vi "Status Monitor (Single Unit).vi"(9 "Update Status Event":refnum<user-event>, 10 "Device Index":i32, 11 "configuration file path":path) -> ()   [LabVIEW 2017, in "Status Monitor Library.lvlib"]
doc: "Connects to the status port and frequently reads the buffer. \n\nAttempts to decode that data in a status message. If the decoding is sucessful, a user event is triggered and that status message is made available through the event."
uses:
  Status Monitor Library.lvlib
  Combined Status and Transient/SubVIs/Device Status and Index--Cluster.ctl
  Communications/Typedefs/DTACQ Module Carrier Status.ctl
  Communications/Typedefs/DTACQ Status--Enum.ctl
  Communications/Communications Library.lvlib
panel:
  in  "Stop":bool
  out "Demuxing":bool
  out "Total Samples":i32
  out "Post-Buffered Samples":i32
  out "Pre-Buffered Samples":i32
  out "Device State":T1(ring)
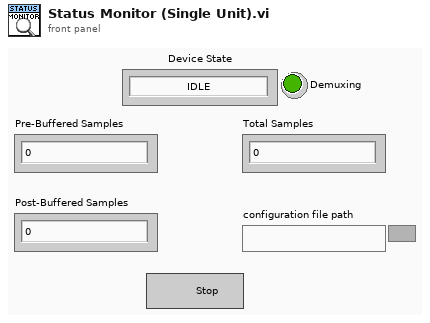
[diagram p1: front panel]
types:
  T1 = enum16{"IDLE", "ARM", "RUN_PRE-TRIGGER", "RUN_POST-TRIGGER", "POST_PROCESS", "CLEANUP"}
  T2 = typedef "Communications Library.lvlib/DTACQ Module Carrier Configuration--Cluster.ctl" = cluster{"Name":string, "IP":string, "Control Port":i32, "Timeout (ms)":i32, "Continuous Capture Port (Multiplexed)":i32, "Start HIL Shot Port":i32, "AWG Upload Port (Multiplexed)":i32, "Download Captured Data Port (Multiplexed)":i32, "Module Slots":i32, "Module Configurations":T3[]}
  T3 = typedef "Communications Library.lvlib/DTACQ Module Configuration--Cluster.ctl" = cluster{"Name":string, "Position":string, "Module Type":T4, "Control Port":i32, "Timeout (ms)":i32, "Channels":i32}
  T4 = typedef "Communications Library.lvlib/DTACQ Device Type--Enum.ctl" = enum16{"Carrier", "Analog In Module", "Analog Out Module", "Generic Module"}
  T5 = typedef "Communications Library.lvlib/DTACQ Connection Data--Cluster.ctl" = cluster{"Description":string, "Address":string, "Port":u16, "timeout (ms)":i32, "Termination Character":string, "TCP Connection Reference":refnum<k5>, "Open Connection":bool}
  T6 = typedef "Device Status and Index--Cluster.ctl" = cluster{"Device Index":i32, "Module Carrier Status":T7}
  T7 = typedef "Communications Library.lvlib/DTACQ Module Carrier Status.ctl" = cluster{"DTACQ State":T8, "Pre-Trigger Samples":i32, "Post-Trigger Samples":i32, "Total Samples":i32, "Post Processing":bool}
  T8 = typedef "Communications Library.lvlib/DTACQ Status--Enum.ctl" = enum16{"IDLE", "ARM", "RUN_PRE-TRIGGER", "RUN_POST-TRIGGER", "POST_PROCESS", "CLEANUP"}
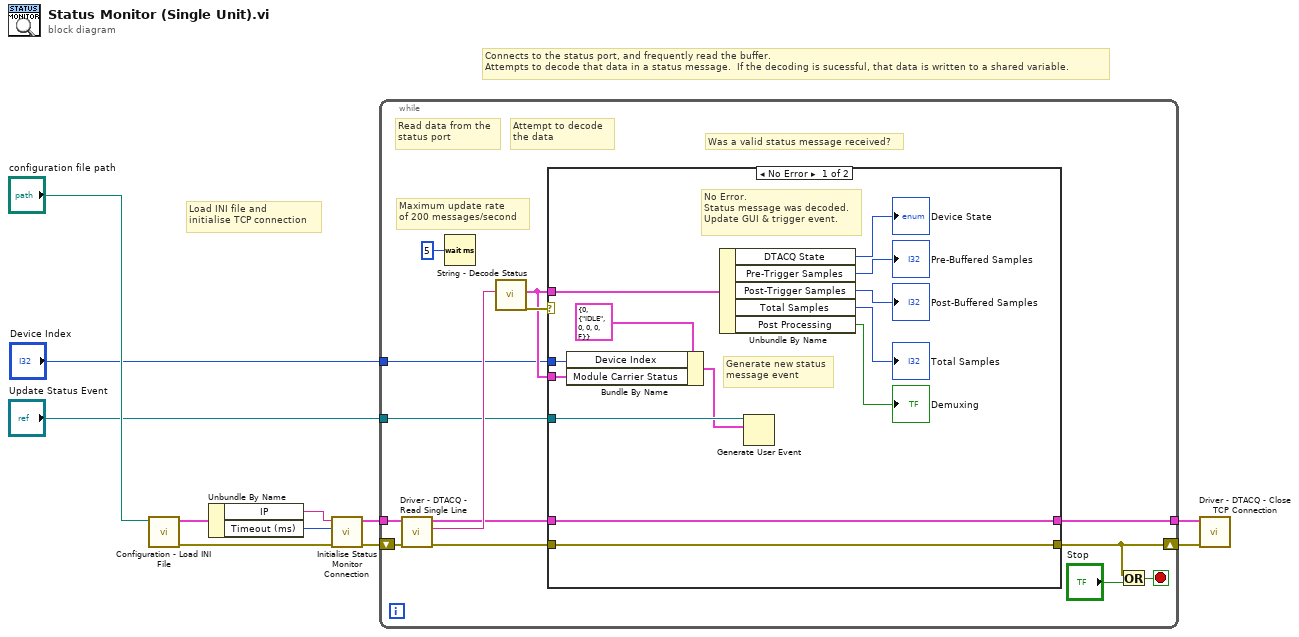
[diagram p0: block diagram]
diagram:
  # "Connects to the status port, and frequently read the buffer.  \nAttempts to decode that data in a status message.  If the decoding is sucessful, that data is written to a shared variable."
  # "Load INI file and\ninitialise TCP connection"
  n1 = call "Configuration - Load INI File.vi"("configuration file path"="configuration file path") -> ("error out"=w6:errorcluster, "Carrier Configuration Out"=w8:T2)  [unwired: 9 in]
  n2 = Unbundle By Name(w8) -> ("IP"=w7:string, "Timeout (ms)"=w5:i32)
  n3 = call "Initialise Status Monitor Connection.vi"("error in"=w6, "timeout (ms)"=w5, "Address"=w7) -> ("error out"=w3:errorcluster, "Status Connection Out"=w11:T5)  [unwired: 7 in]
  n4 = while {
    tunnel: w11 -> [w25]
    shift-right: [w16] -> w10
    shift-left: w3 -> [w23]
    tunnel: [w14] -> w9
    tunnel: "Update Status Event" -> [w13]
    tunnel: "Device Index" -> [w12]
    stop <- w21 stop-if-true
    # "Was a valid status message received?"
    # "Attempt to decode\nthe data"
    # "Read data from the\nstatus port"
    # "Maximum update rate\nof 200 messages/second"
    n5 = call "Driver - DTACQ - Read Single Line.vi"("error in"=w23, "DTACQ Connection Data In"=w25) -> ("error out"=w17:errorcluster, "Read String"=w24:string, "DTACQ Connection Data Out"=w15:T5)  [unwired: 6 in, 1 out]
    n6 = Wait (ms)(milliseconds to wait=u32 5) -> ()  [unwired: 1 out]
    n7 = call "String - Decode Status.vi"("Status Response String"=w24) -> ("error out"=w22:errorcluster, "Module Carrier Status"=w18:T7)  [unwired: 9 in]
    n8 = case shown="No Error" w22 {
      tunnel: w18 -> [w31 _]
      tunnel: w18 -> [w26 _]
      tunnel: w17 -> [w30 w40]
      tunnel: [w30 w40] -> w16
      tunnel: w15 -> [w33 w39]
      tunnel: [w33 w39] -> w14
      tunnel: w13 -> [w32 _]
      tunnel: w12 -> [w28 _]
      frame No Error {
        # "Generate new status\nmessage event"
        # "No Error.\nStatus message was decoded.\nUpdate GUI & trigger event."
        n9 = Bundle By Name(cluster=T6 {"Device Index"=0, "Module Carrier Status"={"DTACQ State"=enum."IDLE", "Pre-Trigger Samples"=0, "Post-Trigger Samples"=0, "Total Samples"=0, "Post Processing"=FALSE}} ("Device Status and Index"), "Device Index"=w28, "Module Carrier Status"=w26) -> (w27:T6)
        n10 = Unbundle By Name(w31) -> ("DTACQ State"=→"Device State":T8, "Pre-Trigger Samples"=→"Pre-Buffered Samples":i32, "Post-Trigger Samples"=→"Post-Buffered Samples":i32, "Total Samples"=→"Total Samples":i32, "Post Processing"=→"Demuxing":bool)
        n11 = Generate User Event(user event=w32, event data cluster=w27) -> ()  [unwired: 2 in, 2 out]
      }
      frame Error {
        # "Error decoding message.\nNot a valid status message,\nso leave the GUI as-is."
      }
    }
    n12 = Or(x=w16, y="Stop") -> (x .or. y?=w21:bool)
  }
  n13 = call "Driver - DTACQ - Close TCP Connection.vi"("error in"=w10, "DTACQ Connection Data In"=w9) -> ()  [unwired: 8 in, 2 out]
